vi "Vending Machine.vi"() -> ()   [LabVIEW 2016]
panel:
  in  "반환":bool
  out "거스름돈":string
  out "백원 갯수":string
  out "오백원 갯수":string
  in  "500원권":bool
  out "파워":dbl(slide)
  out "비타민":dbl(slide)
  out "파워에이드 재고":string
  out "비타민 워터 재고":string
  out "사이다 재고":string
  out "콜라 재고":string
  out "Display \nMoney":dbl
  out "사이다 뽑음":dbl(slide)
  in  "100원권":bool
  in  "1000원권":bool
  in  "5000원권":bool
  in  "10000원권":bool
  in  "카드":bool
  in  "2000 원":bool
  in  "1500 원":bool
  in  "1000 원":bool
  in  "700 원":bool
  in  "자판기 멈춤":bool
  out "콜라뽑음":dbl(slide)
  # "27기 인턴 \n 하 유 진"
  # "원"
  # "거스름 동전 재고"
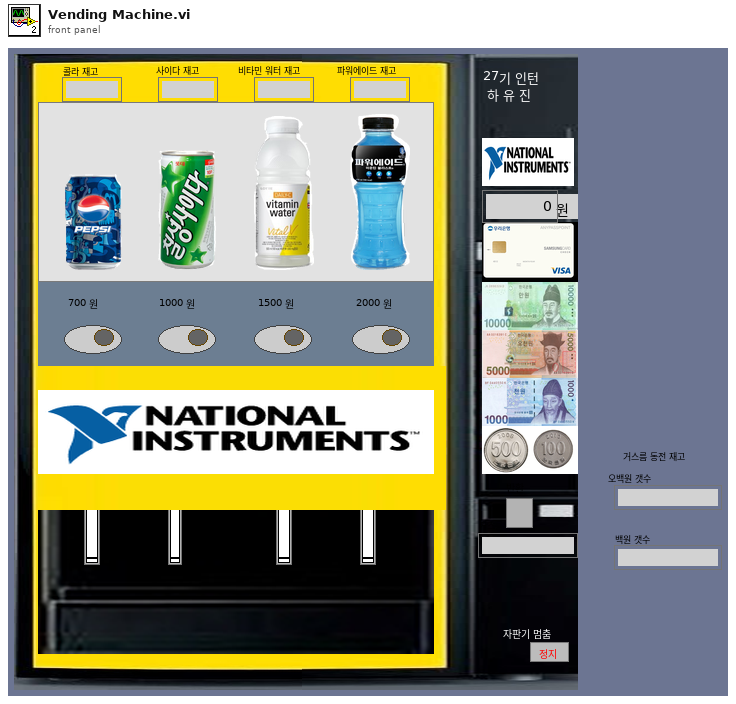
[diagram p1: front panel]
types:
  T1 = cluster{"재고1":i32, "재고2":i32, "재고3":i32, "재고4":i32}
  T2 = cluster{"700원":bool, " 1000원":bool, "1500원":bool, "2000원":bool}
  T3 = cluster{"10000":bool, " 5000":bool, "1000":bool, "100":bool, "500":bool, "카드":bool}
  T4 = typedef "컨트롤 3.ctl" = enum32{"대기", "돈 투입", "돈 반환", "음료 재고", "음료 주문", "카드"}
  T5 = enum16{"대기", "돈 투입", "돈 반환", "음료 재고", "음료 주문", "카드"}
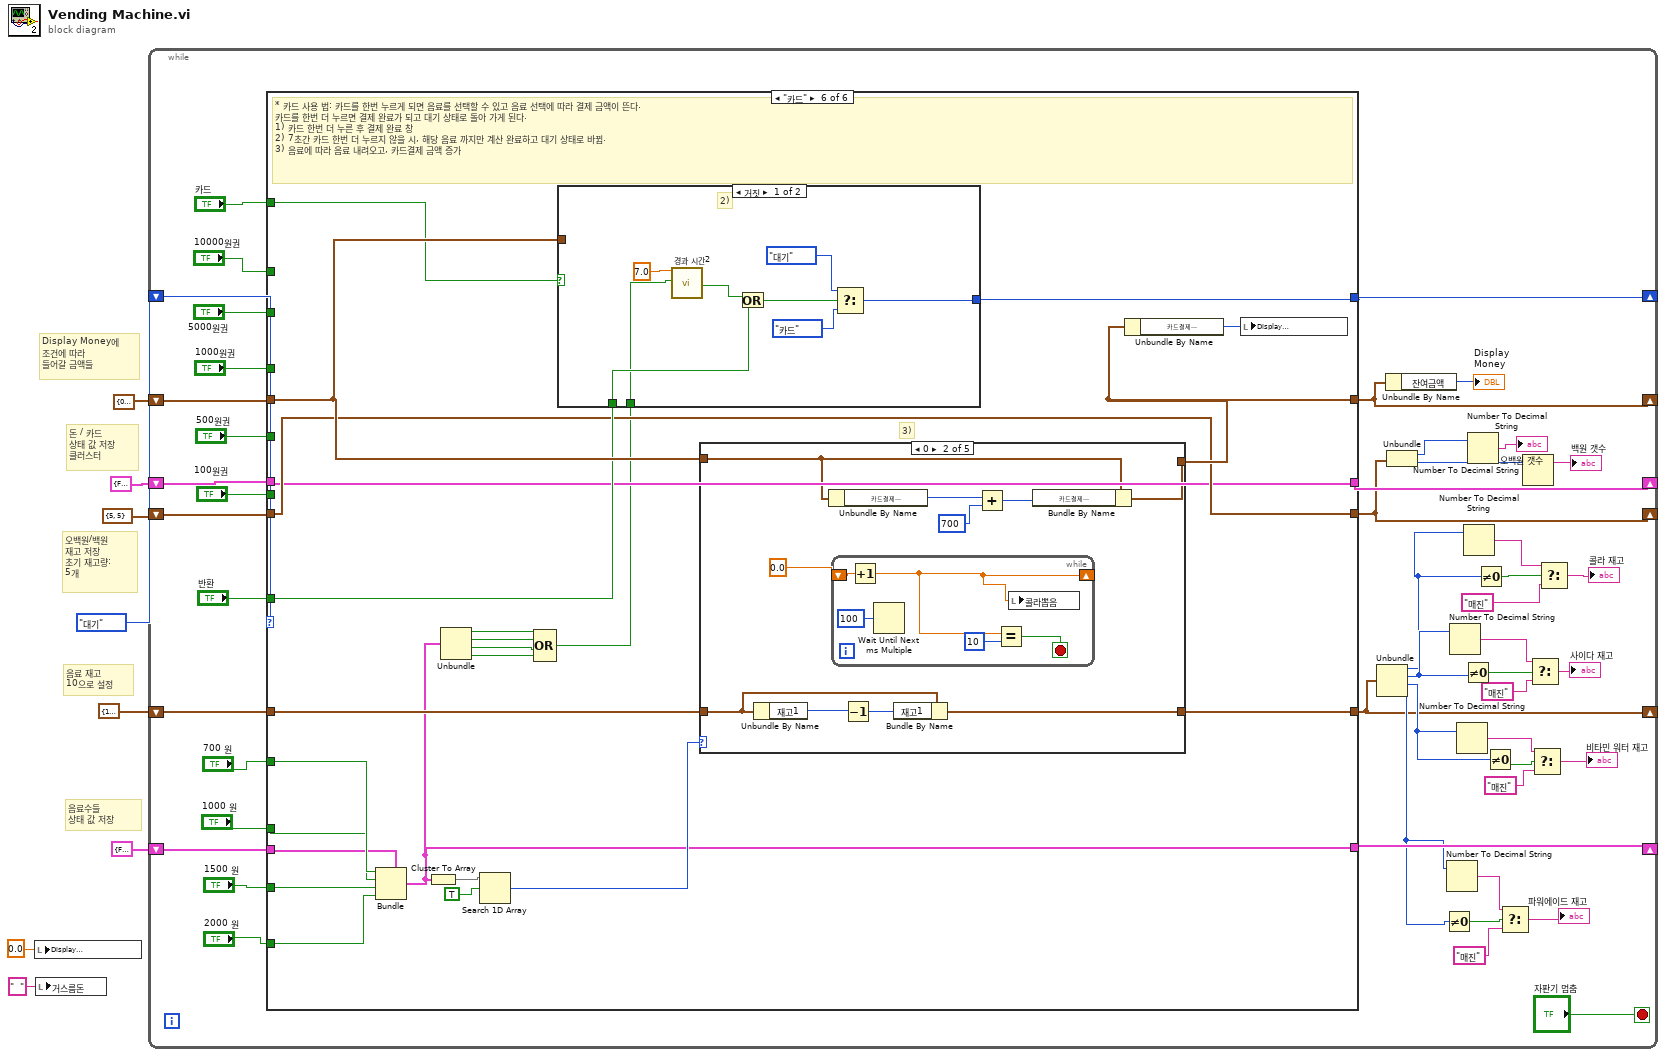
[diagram p0: block diagram]
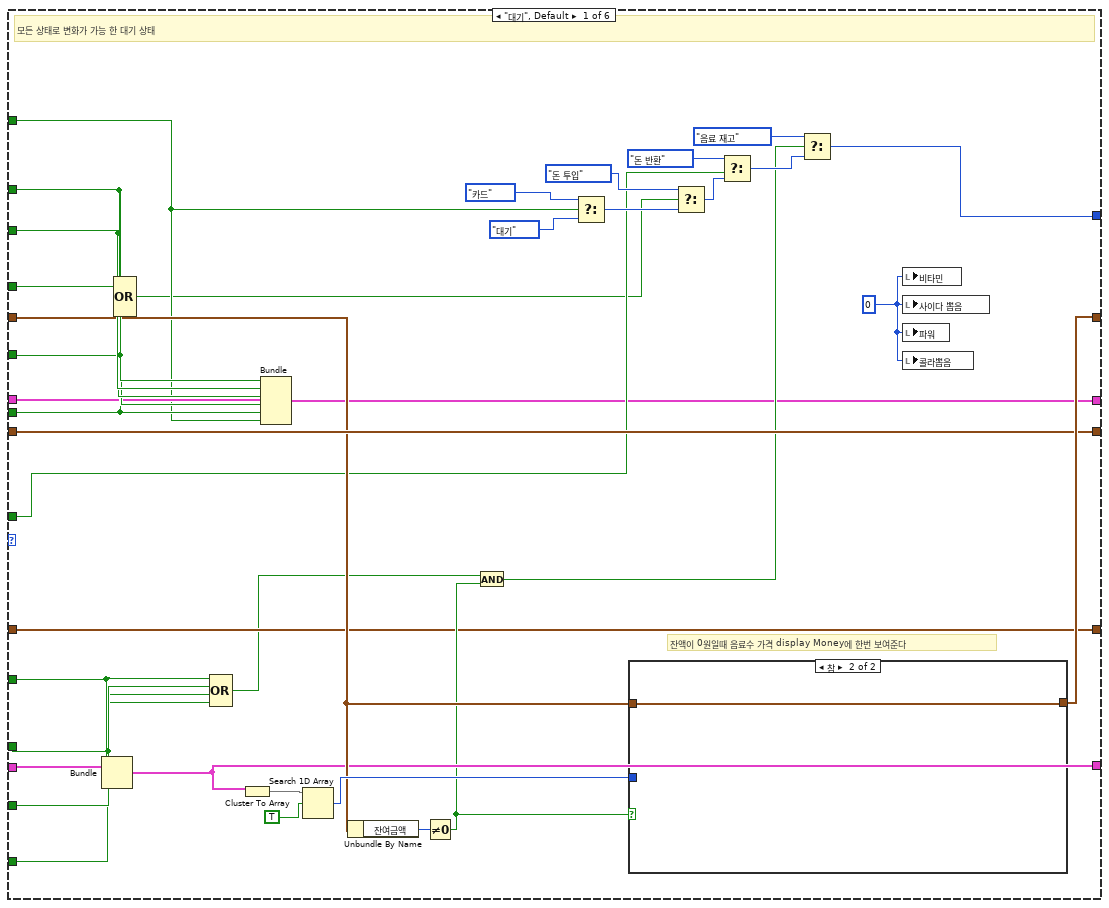
[diagram p2: hidden frame]
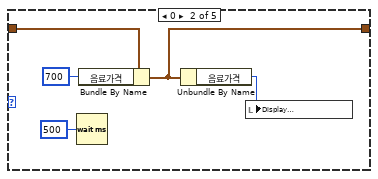
[diagram p4: hidden frame]
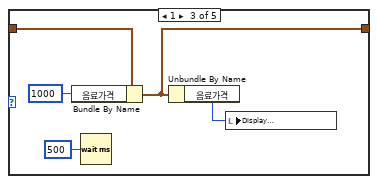
[diagram p5: hidden frame]
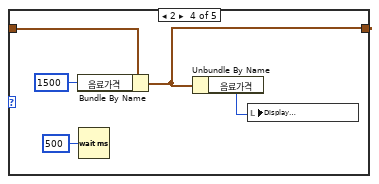
[diagram p6: hidden frame]
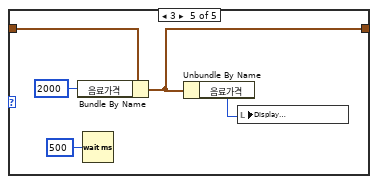
[diagram p7: hidden frame]
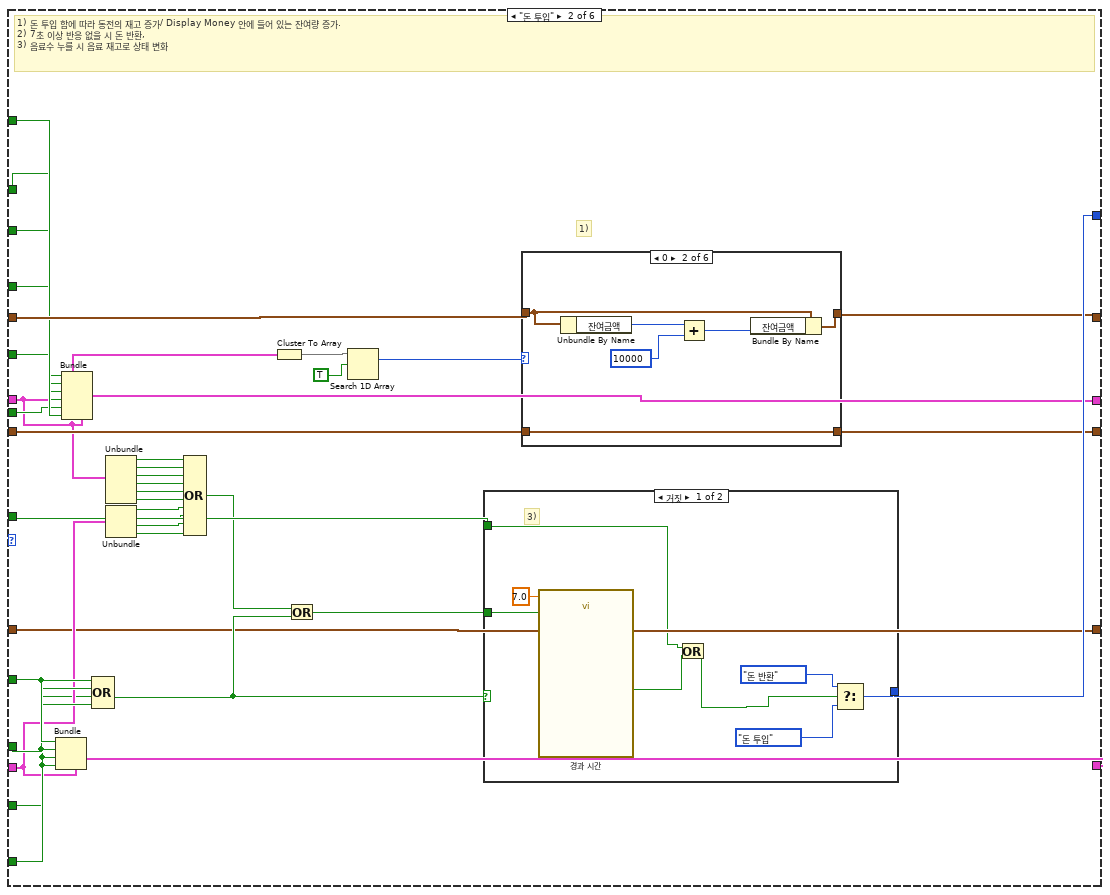
[diagram p8: hidden frame]
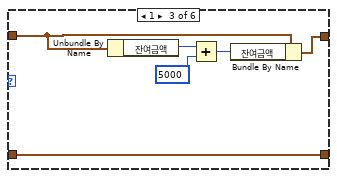
[diagram p10: hidden frame]
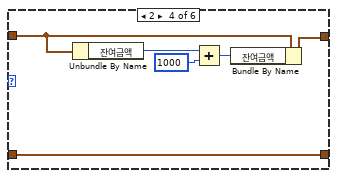
[diagram p11: hidden frame]
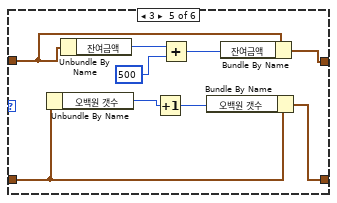
[diagram p12: hidden frame]
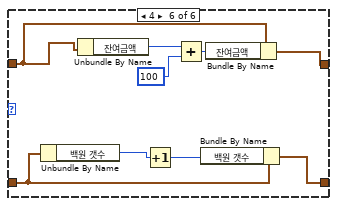
[diagram p13: hidden frame]
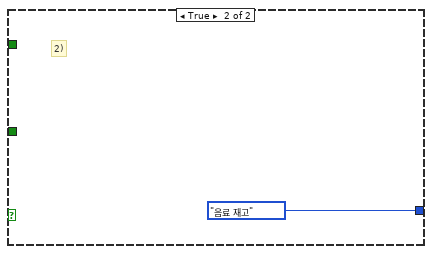
[diagram p14: hidden frame]
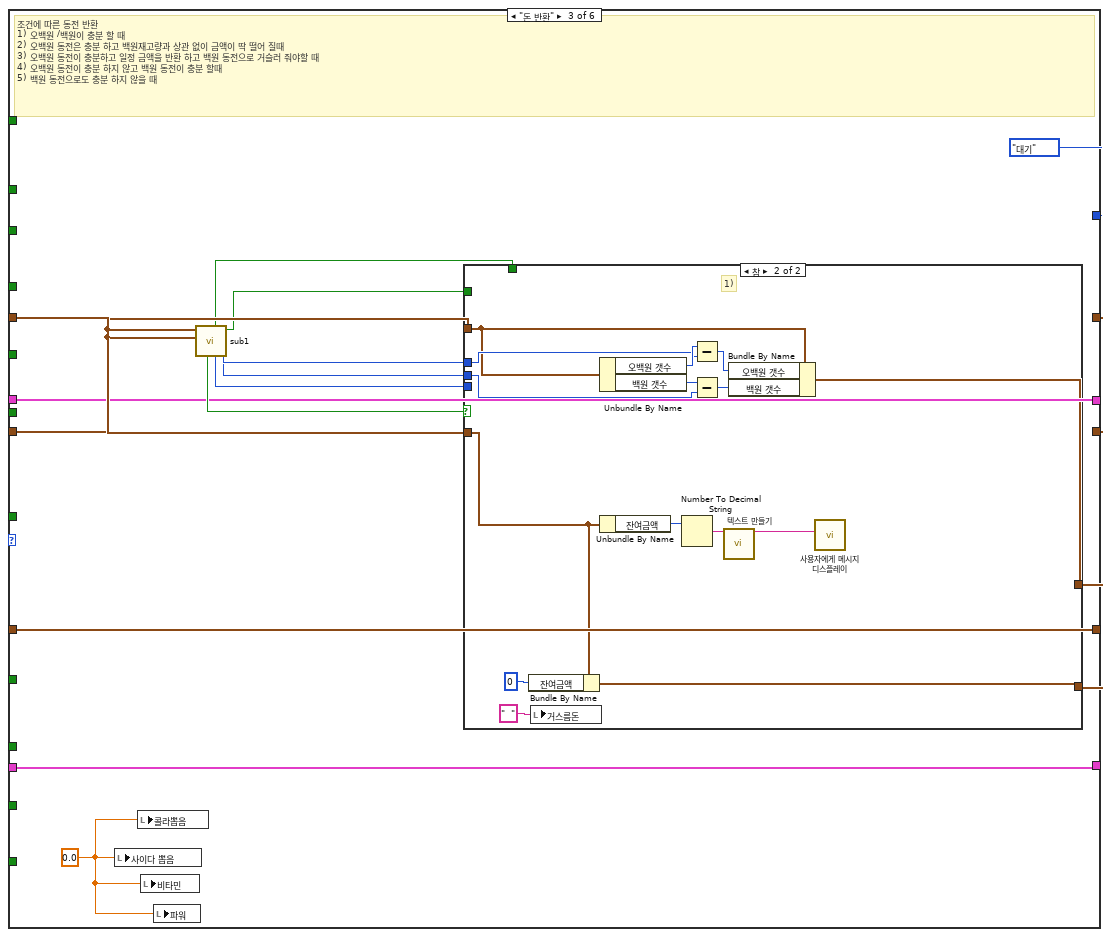
[diagram p15: hidden frame]
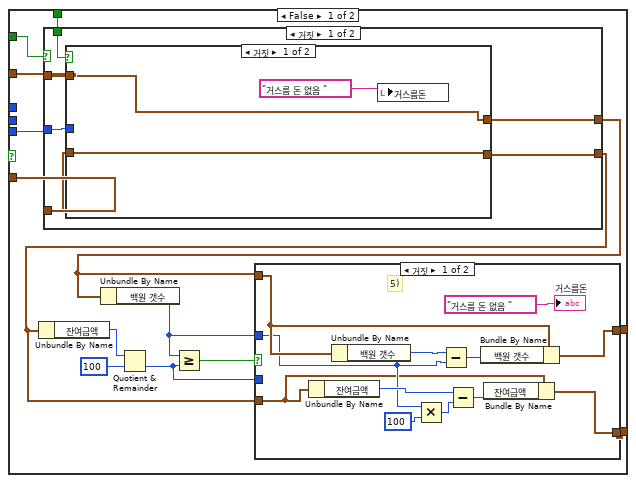
[diagram p16: hidden frame]
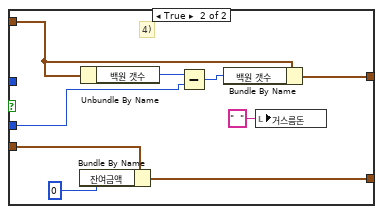
[diagram p17: hidden frame]
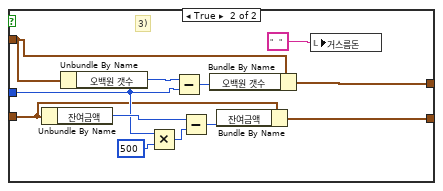
[diagram p18: hidden frame]
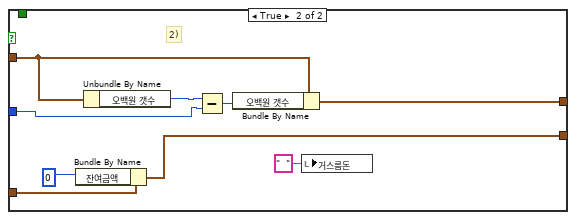
[diagram p19: hidden frame]
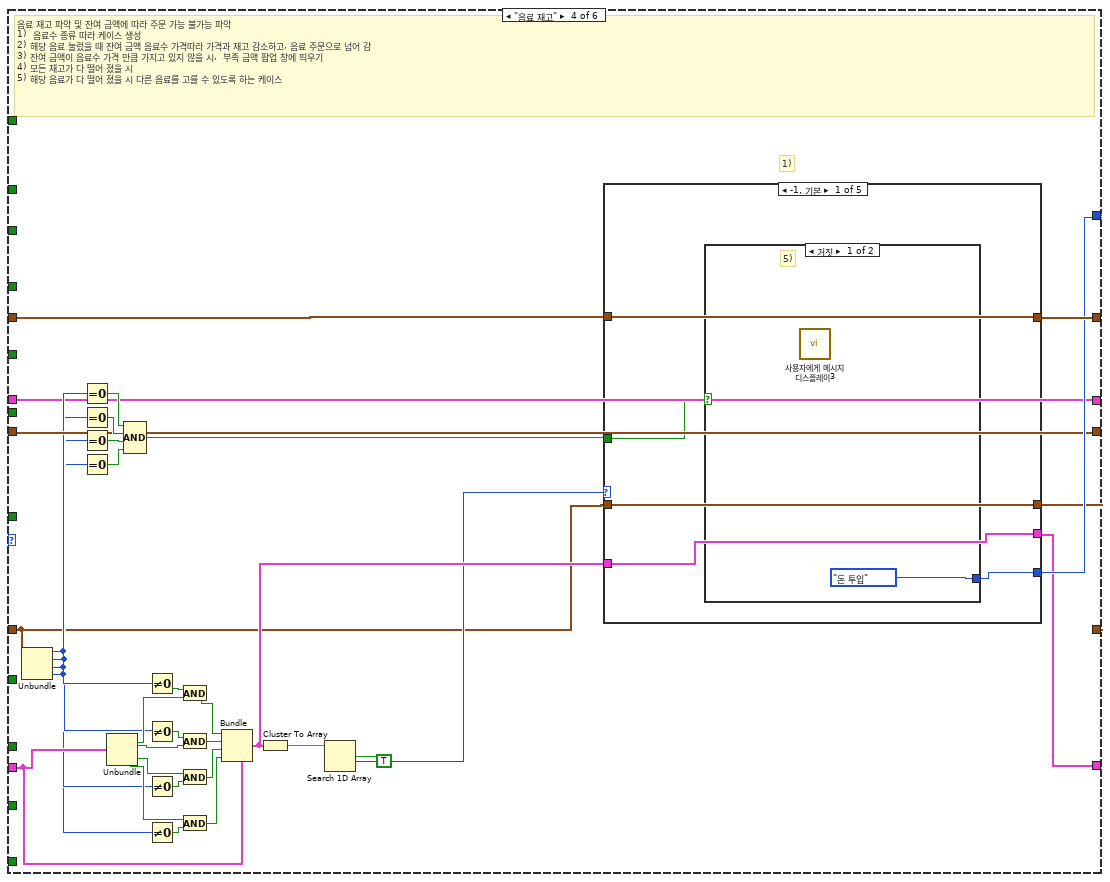
[diagram p20: hidden frame]
diagram:
  # "음료 재고 \n10으로 설정"
  # "음료수들  \n상태 값 저장"
  # "오백원/백원\n재고 저장\n초기 재고량: \n5개"
  # "돈 / 카드 \n상태 값 저장\n클러스터"
  # "Display Money에 \n조건에 따라\n들어갈 금액들"
  n1 = local write "Display \nMoney"(0.0 ("Display \nMoney")) -> ()
  n2 = local write "거스름돈"("  " ("거스름돈")) -> ()
  n3 = while {
    shift-right: [w50] -> _
    shift-left: 컨트롤_3."대기" -> [w39]
    shift-right: [w42] -> _
    shift-left: cluster{"잔여금액":i32, "카드결제\n금액":i32, "음료가격":i32} {"잔여금액"=0, "카드결제\n금액"=0, "음료가격"=0} -> [w45]
    shift-right: [w44] -> _
    shift-left: T3 {"10000"=FALSE, " 5000"=FALSE, "1000"=FALSE, "100"=FALSE, "500"=FALSE, "카드"=FALSE} -> [w38]
    shift-right: [w40] -> _
    shift-left: T2 {"700원"=FALSE, " 1000원"=FALSE, "1500원"=FALSE, "2000원"=FALSE} -> [w43]
    shift-right: [w10] -> _
    shift-left: cluster{"오백원 갯수":i32, " 백원 갯수":i32} {"오백원 갯수"=5, " 백원 갯수"=5} -> [w24]
    shift-right: [w13] -> _
    shift-left: T1 {"재고1"=10, "재고2"=10, "재고3"=10, "재고4"=10} -> [w19]
    stop <- "자판기 멈춤" stop-if-true
    n4 = case shown="\"카드\"" w39 {
      tunnel: "카드" -> [w72 w146 _ _ _ w519]
      tunnel: "10000원권" -> [w94 w142 _ _ _ _]
      tunnel: "5000원권" -> [w93 w141 _ _ _ _]
      tunnel: "1000원권" -> [w92 w140 _ _ _ _]
      tunnel: "500원권" -> [w91 w139 _ _ _ _]
      tunnel: "100원권" -> [w90 w138 _ _ _ _]
      tunnel: [w65 w156 T5."대기" w314 w468 w525] -> w50
      tunnel: "700 원" -> [w80 w155 _ _ _ w534]
      tunnel: "1000 원" -> [w79 w154 _ _ _ w533]
      tunnel: "1500 원" -> [w78 w120 _ _ _ w532]
      tunnel: "2000 원" -> [w77 w153 _ _ _ w531]
      tunnel: w45 -> [w81 w148 w217 w315 w480 w527]
      tunnel: [w85 w147 w206 w317 w480 w524] -> w42
      tunnel: w38 -> [w84 w135 w204 w300 w483 w518]
      tunnel: [w61 w121 w204 w300 w483 w518] -> w44
      tunnel: w43 -> [w86 w128 w205 w324 w482 w517]
      tunnel: [w76 w152 w205 w299 w482 w516] -> w40
      tunnel: "반환" -> [w63 w145 _ _ w474 w526]
      tunnel: w24 -> [w82 w144 w215 w307 w481 w522]
      tunnel: [w82 w143 w216 w307 w481 w522] -> w10
      tunnel: w19 -> [w59 w122 w207 w302 w478 w521]
      tunnel: [w59 w122 w207 w301 w478 w520] -> w13
      frame "대기", Default {
        w83 = 0
        # "잔액이 0원일때 음료수 가격 display Money에 한번 보여준다"
        # "모든 상태로 변화가 가능 한 대기 상태"
        n5 = Bundle(cluster=w86, "700원"=w80, "1000원"=w79, "1500원"=w78, "2000원"=w77) -> (w76:T2)
        n6 = Compound Arithmetic op=OR ("복합 연산")(w94, w93, w92, w91, w90) -> (w62:bool)
        n7 = Compound Arithmetic op=OR ("복합 연산")(w80, w79, w78, w77) -> (w58:bool)
        n8 = Cluster To Array(cluster=w76) -> (array=w89:bool[])
        n9 = Bundle(cluster=w84, "10000"=w94, "5000"=w93, "1000"=w92, "100"=w91, "500"=w90, "카드"=w72) -> (w61:T3)
        n10 = Search 1D Array(1D array=w89, element=TRUE ("원소")) -> (index of element=w88:i32)  [unwired: 1 in]
        n11 = Unbundle By Name(w81) -> ("잔여금액"=w60:i32)
        n12 = Not Equal To 0?(x=w60) -> (x != 0?=w75:bool)
        n13 = And(x=w58, y=w75) -> (x .and. y?=w67:bool)
        n14 = Select(t=T5."카드", s=w72, f=T5."대기") -> (s? t:f=w71:T5)
        n15 = case shown="참" w75 {
          tunnel: w88 -> [w97 _]
          tunnel: [w96 w119] -> w85
          tunnel: w81 -> [w95 w119]
          frame False {
            n16 = case shown="-1, 기본" w97 {
              tunnel: w95 -> [w98 w103 w107 w112 w117]
              tunnel: [w98 w101 w105 w110 w115] -> w96
              frame -1, Default {
              }
              frame 0 {
                n17 = Wait (ms)(milliseconds to wait=u32 500 ("대기 시간 (ms)")) -> ()  [unwired: 1 out]
                n18 = Bundle By Name(cluster=w103, "음료가격"=700 ("잔여금액")) -> (w101:cluster{"잔여금액":i32, "카드결제\n금액":i32, "음료가격":i32})
                n19 = Unbundle By Name(w101) -> ("음료가격"=w100:i32)
                n20 = local write "Display \nMoney"(w100) -> ()
              }
              frame 1 {
                n21 = Bundle By Name(cluster=w107, "음료가격"=1000 ("잔여금액")) -> (w105:cluster{"잔여금액":i32, "카드결제\n금액":i32, "음료가격":i32})
                n22 = Wait (ms)(milliseconds to wait=u32 500 ("대기 시간 (ms)")) -> ()  [unwired: 1 out]
                n23 = Unbundle By Name(w105) -> ("음료가격"=w106:i32)
                n24 = local write "Display \nMoney"(w106) -> ()
              }
              frame 2 {
                n25 = Bundle By Name(cluster=w112, "음료가격"=1500 ("잔여금액")) -> (w110:cluster{"잔여금액":i32, "카드결제\n금액":i32, "음료가격":i32})
                n26 = Wait (ms)(milliseconds to wait=u32 500 ("대기 시간 (ms)")) -> ()  [unwired: 1 out]
                n27 = Unbundle By Name(w110) -> ("음료가격"=w111:i32)
                n28 = local write "Display \nMoney"(w111) -> ()
              }
              frame 3 {
                n29 = Bundle By Name(cluster=w117, "음료가격"=2000 ("잔여금액")) -> (w115:cluster{"잔여금액":i32, "카드결제\n금액":i32, "음료가격":i32})
                n30 = Wait (ms)(milliseconds to wait=u32 500 ("대기 시간 (ms)")) -> ()  [unwired: 1 out]
                n31 = Unbundle By Name(w115) -> ("음료가격"=w116:i32)
                n32 = local write "Display \nMoney"(w116) -> ()
              }
            }
          }
          frame True {
          }
        }
        n33 = Select(t=T5."돈 투입", s=w62, f=w71) -> (s? t:f=w69:T5)
        n34 = Select(t=T5."돈 반환", s=w63, f=w69) -> (s? t:f=w68:T5)
        n35 = Select(t=T5."음료 재고", s=w67, f=w68) -> (s? t:f=w65:T5)
        n36 = local write "비타민"(w83) -> ()
        n37 = local write "사이다 뽑음"(w83) -> ()
        n38 = local write "파워"(w83) -> ()
        n39 = local write "콜라뽑음"(w83) -> ()
      }
      frame "돈 투입" {
        # "1)"
        # "1) 돈 투입 함에 따라 동전의 재고 증가/ Display Money 안에 들어 있는 잔여량 증가.\n2) 7초 이상 반응 없을 시 돈 반환, \n3) 음료수 누를 시 음료 재고로 상태 변화"
        n40 = Bundle(cluster=w128, "700원"=w155, "1000원"=w154, "1500원"=w120, "2000원"=w153) -> (w152:T2)
        n41 = Bundle(cluster=w135, "10000"=w142, "5000"=w141, "1000"=w140, "100"=w139, "500"=w138, "카드"=w146) -> (w121:T3)
        n42 = Compound Arithmetic op=OR ("복합 연산")(w155, w154, w120, w153) -> (w123:bool)
        n43 = Unbundle(w135) -> ("10000"=w134:bool, "5000"=w133:bool, "1000"=w132:bool, "100"=w131:bool, "500"=w130:bool, "카드"=w129:bool)
        n44 = Unbundle(w128) -> ("700원"=w127:bool, "1000원"=w126:bool, "1500원"=w125:bool, "2000원"=w124:bool)
        n45 = Compound Arithmetic op=OR ("복합 연산")(w134, w133, w132, w131, w130, w129, w127, w126, w125, w124) -> (w137:bool)
        n46 = Cluster To Array(cluster=w135) -> (array=w151:bool[])
        n47 = Or(x=w137, y=w123) -> (x .or. y?=w136:bool)
        n48 = Search 1D Array(1D array=w151, element=TRUE ("원소")) -> (index of element=w149:i32)  [unwired: 1 in]
        n49 = case shown="거짓" w123 {
          tunnel: [w201 T5."음료 재고"] -> w156
          tunnel: w145 -> [w199 _]
          tunnel: w136 -> [w195 _]
          frame False {
            # "3)"
            n50 = call "경과 시간"("Time Target (s)"=7.0, "Reset"=w195) -> ("Time has Elapsed"=w196:bool)  [unwired: 10 in, 7 out]
            n51 = Or(x=w199, y=w196) -> (x .or. y?=w198:bool)
            n52 = Select(t=T5."돈 반환", s=w198, f=T5."돈 투입") -> (s? t:f=w201:T5)
          }
          frame True {
            # "2)"
          }
        }
        n53 = case shown="0" w149 {
          tunnel: w148 -> [w158 w161 w167 w173 w182 w191]
          tunnel: [w158 w160 w166 w172 w181 w190] -> w147
          tunnel: w144 -> [w157 w159 w165 w171 w179 w187]
          tunnel: [w157 w159 w165 w171 w178 w186] -> w143
          frame -1, Default {
          }
          frame 0 {
            n54 = Unbundle By Name(w161) -> ("잔여금액"=w162:i32)
            n55 = Add(x=w162, y=10000) -> (x+y=w164:i32)
            n56 = Bundle By Name(cluster=w161, "잔여금액"=w164) -> (w160:cluster{"잔여금액":i32, "카드결제\n금액":i32, "음료가격":i32})
          }
          frame 1 {
            n57 = Unbundle By Name(w167) -> ("잔여금액"=w168:i32)
            n58 = Add(x=w168, y=5000) -> (x+y=w169:i32)
            n59 = Bundle By Name(cluster=w167, "잔여금액"=w169) -> (w166:cluster{"잔여금액":i32, "카드결제\n금액":i32, "음료가격":i32})
          }
          frame 2 {
            n60 = Unbundle By Name(w173) -> ("잔여금액"=w174:i32)
            n61 = Add(x=w174, y=1000) -> (x+y=w176:i32)
            n62 = Bundle By Name(cluster=w173, "잔여금액"=w176) -> (w172:cluster{"잔여금액":i32, "카드결제\n금액":i32, "음료가격":i32})
          }
          frame 3 {
            n63 = Unbundle By Name(w179) -> ("오백원 갯수"=w177:i32)
            n64 = Unbundle By Name(w182) -> ("잔여금액"=w184:i32)
            n65 = Increment(x=w177) -> (x+1=w180:i32)
            n66 = Add(x=w184, y=500) -> (x+y=w185:i32)
            n67 = Bundle By Name(cluster=w179, "오백원 갯수"=w180) -> (w178:cluster{"오백원 갯수":i32, " 백원 갯수":i32})
            n68 = Bundle By Name(cluster=w182, "잔여금액"=w185) -> (w181:cluster{"잔여금액":i32, "카드결제\n금액":i32, "음료가격":i32})
          }
          frame 4 {
            n69 = Unbundle By Name(w187) -> ("백원 갯수"=w188:i32)
            n70 = Unbundle By Name(w191) -> ("잔여금액"=w192:i32)
            n71 = Increment(x=w188) -> (x+1=w189:i32)
            n72 = Add(x=w192, y=100) -> (x+y=w194:i32)
            n73 = Bundle By Name(cluster=w187, "백원 갯수"=w189) -> (w186:cluster{"오백원 갯수":i32, " 백원 갯수":i32})
            n74 = Bundle By Name(cluster=w191, "잔여금액"=w194) -> (w190:cluster{"잔여금액":i32, "카드결제\n금액":i32, "음료가격":i32})
          }
        }
      }
      frame "돈 반환" {
        w208 = 0.0 ("사이다 뽑힘")
        # "조건에 따른 동전 반환 \n1) 오백원 /백원이 충분 할 때\n2) 오백원 동전은 충분 하고 백원재고량과 상관 없이 금액이 딱 떨어 질때\n3) 오백원 동전이 충분하고 일정 금액을 반환 하고 백원 동전으로 거슬러 줘야할 때 \n4) 오백원 동전이 충분 하지 않고 백원 동전이 충분 할때\n5) 백원 동전으로도 충분 하지 않을 때"
        n75 = local write "사이다 뽑음"(w208) -> ()
        n76 = local write "콜라뽑음"(w208) -> ()
        n77 = local write "비타민"(w208) -> ()
        n78 = local write "파워"(w208) -> ()
        n79 = call "sub1.vi"("클러스터"=w215, "클러스터 2"=w217) -> ("숫자형"=w212:i32, "숫자형 2"=w213:i32, "불리언 2"=w210:bool, "오백원 갯수"=w211:i32, "불리언"=w209:bool, "불리언 3"=w214:bool)  [unwired: 4 in]
        n80 = case shown="참" w214 {
          tunnel: w215 -> [w231 w296]
          tunnel: w213 -> [_ w297]
          tunnel: w212 -> [_ w293]
          tunnel: w210 -> [w232 _]
          tunnel: w217 -> [w230 w287]
          tunnel: w211 -> [w229 _]
          tunnel: [w223 w286] -> w206
          tunnel: [w222 w285] -> w216
          tunnel: w209 -> [w219 _]
          frame False {
            n81 = case shown="거짓" w232 {
              tunnel: w231 -> [w259 w279]
              tunnel: [w258 w282] -> w225
              tunnel: w229 -> [w257 w281]
              tunnel: w230 -> [w256 w277]
              tunnel: [w255 w276] -> w224
              tunnel: w219 -> [w254 _]
              frame False {
                n82 = case shown="거짓" w254 {
                  tunnel: w259 -> [w261 w272]
                  tunnel: [w261 w271] -> w258
                  tunnel: w257 -> [_ w269]
                  tunnel: w256 -> [w260 w267]
                  tunnel: [w260 w265] -> w255
                  frame False {
                    n83 = local write "거스름돈"("거스름 돈 없음 " ("거스름돈")) -> ()
                  }
                  frame True {
                    # "3)"
                    n84 = Unbundle By Name(w267) -> ("잔여금액"=w270:i32)
                    n85 = Unbundle By Name(w272) -> ("오백원 갯수"=w273:i32)
                    n86 = Multiply(x=w269, y=500) -> (x*y=w264:i32)
                    n87 = Subtract(x=w273, y=w269) -> (x-y=w274:i32)
                    n88 = Subtract(x=w270, y=w264) -> (x-y=w266:i32)
                    n89 = Bundle By Name(cluster=w272, "오백원 갯수"=w274) -> (w271:cluster{"오백원 갯수":i32, " 백원 갯수":i32})
                    n90 = Bundle By Name(cluster=w267, "잔여금액"=w266) -> (w265:cluster{"잔여금액":i32, "카드결제\n금액":i32, "음료가격":i32})
                    n91 = local write "거스름돈"("   " ("거스름돈")) -> ()
                  }
                }
              }
              frame True {
                # "2)"
                n92 = Bundle By Name(cluster=w277, "잔여금액"=0) -> (w276:cluster{"잔여금액":i32, "카드결제\n금액":i32, "음료가격":i32})
                n93 = Unbundle By Name(w279) -> ("오백원 갯수"=w280:i32)
                n94 = Subtract(x=w280, y=w281) -> (x-y=w283:i32)
                n95 = Bundle By Name(cluster=w279, "오백원 갯수"=w283) -> (w282:cluster{"오백원 갯수":i32, " 백원 갯수":i32})
                n96 = local write "거스름돈"("  " ("거스름돈")) -> ()
              }
            }
            n97 = Unbundle By Name(w224) -> ("잔여금액"=w227:i32)
            n98 = Unbundle By Name(w225) -> ("백원 갯수"=w221:i32)
            n99 = Quotient & Remainder(x=w227, y=100) -> (floor(x/y)=w220:i32)  [unwired: 1 out]
            n100 = Greater Or Equal?(x=w221, y=w220) -> (x >= y?=w228:bool)
            n101 = case shown="거짓" w228 {
              tunnel: w225 -> [w237 w250]
              tunnel: w224 -> [w235 w249]
              tunnel: w220 -> [_ w248]
              tunnel: [w234 w247] -> w223
              tunnel: [w233 w246] -> w222
              tunnel: w221 -> [w236 _]
              frame False {
                # "5)"
                n102 = Unbundle By Name(w235) -> ("잔여금액"=w241:i32)
                n103 = Unbundle By Name(w237) -> ("백원 갯수"=w242:i32)
                n104 = Multiply(x=w236, y=100) -> (x*y=w238:i32)
                n105 = Subtract(x=w242, y=w236) -> (x-y=w243:i32)
                n106 = Subtract(x=w241, y=w238) -> (x-y=w239:i32)
                n107 = Bundle By Name(cluster=w237, "백원 갯수"=w243) -> (w233:cluster{"오백원 갯수":i32, " 백원 갯수":i32})
                n108 = Bundle By Name(cluster=w235, "잔여금액"=w239) -> (w234:cluster{"잔여금액":i32, "카드결제\n금액":i32, "음료가격":i32})
                "거스름돈" <- "거스름 돈 없음 " ("거스름돈")
              }
              frame True {
                # "4)"
                n109 = Bundle By Name(cluster=w249, "잔여금액"=0) -> (w247:cluster{"잔여금액":i32, "카드결제\n금액":i32, "음료가격":i32})
                n110 = Unbundle By Name(w250) -> ("백원 갯수"=w253:i32)
                n111 = Subtract(x=w253, y=w248) -> (x-y=w252:i32)
                n112 = Bundle By Name(cluster=w250, "백원 갯수"=w252) -> (w246:cluster{"오백원 갯수":i32, " 백원 갯수":i32})
                n113 = local write "거스름돈"("  " ("거스름돈")) -> ()
              }
            }
          }
          frame True {
            # "1)"
            n114 = Bundle By Name(cluster=w287, "잔여금액"=0) -> (w286:cluster{"잔여금액":i32, "카드결제\n금액":i32, "음료가격":i32})
            n115 = local write "거스름돈"("  " ("거스름돈")) -> ()
            n116 = Unbundle By Name(w296) -> ("오백원 갯수"=w298:i32, "백원 갯수"=w294:i32)
            n117 = Unbundle By Name(w287) -> ("잔여금액"=w289:i32)
            n118 = Number To Decimal String(number=w289) -> (decimal integer string=w291:string)  [unwired: 1 in]
            n119 = Subtract(x=w298, y=w297) -> (x-y=w295:i32)
            n120 = Subtract(x=w294, y=w293) -> (x-y=w292:i32)
            n121 = call "텍스트 만들기"("Beginning Text"=w291) -> ("Result"=w290:string)  [unwired: 13 in, 1 out]
            n122 = Bundle By Name(cluster=w296, "오백원 갯수"=w295, "백원 갯수"=w292) -> (w285:cluster{"오백원 갯수":i32, " 백원 갯수":i32})
            n123 = call "사용자에게 메시지 디스플레이"("Message"=w290) -> ()  [unwired: 9 in, 2 out]
          }
        }
      }
      frame "음료 재고" {
        # "1)"
        # "음료 재고 파악 및 잔여 금액에 따라 주문 가능 불가능 파악\n1)  음료수 종류 따라 케이스 생성\n2) 해당 음료 눌렀을 때 잔여 금액 음료수 가격따라 가격과 재고 감소하고, 음료 주문으로 넘어 감\n3) 잔여 금액이 음료수 가격 만큼 가지고 있지 않을 시,  부족 금액 팝업 창에 띄우기 \n4) 모든 재고가 다 떨어 졌을 시 \n5) 해당 음료가 다 떨어 졌을 시 다른 음료를 고를 수 있도록 하는 케이스"
        n124 = Unbundle(w302) -> ("재고1"=w306:i32, "재고2"=w305:i32, "재고3"=w304:i32, "재고4"=w303:i32)
        n125 = Equal To 0?(x=w306) -> (x = 0?=w312:bool)
        n126 = Equal To 0?(x=w305) -> (x = 0?=w311:bool)
        n127 = Equal To 0?(x=w304) -> (x = 0?=w310:bool)
        n128 = Equal To 0?(x=w303) -> (x = 0?=w309:bool)
        n129 = Unbundle(w324) -> ("700원"=w332:bool, "1000원"=w331:bool, "1500원"=w330:bool, "2000원"=w329:bool)
        n130 = Compound Arithmetic op=AND ("복합 연산")(w312, w311, w310, w309) -> (w308:bool)
        n131 = Not Equal To 0?(x=w306) -> (x != 0?=w328:bool)
        n132 = Not Equal To 0?(x=w305) -> (x != 0?=w325:bool)
        n133 = Not Equal To 0?(x=w304) -> (x != 0?=w326:bool)
        n134 = Not Equal To 0?(x=w303) -> (x != 0?=w327:bool)
        n135 = And(x=w328, y=w332) -> (x .and. y?=w323:bool)
        n136 = And(x=w325, y=w331) -> (x .and. y?=w322:bool)
        n137 = And(x=w330, y=w326) -> (x .and. y?=w321:bool)
        n138 = And(x=w329, y=w327) -> (x .and. y?=w320:bool)
        n139 = Bundle(cluster=w324, "700원"=w323, "1000원"=w322, "1500원"=w321, "2000원"=w320) -> (w316:T2)
        n140 = Cluster To Array(cluster=w316) -> (array=w319:bool[])
        n141 = Search 1D Array(1D array=w319, element=TRUE ("원소")) -> (index of element=w313:i32)  [unwired: 1 in]
        n142 = case shown="-1, 기본" w313 {
          tunnel: w315 -> [w335 w345 w376 w407 w439]
          tunnel: [w335 w349 w381 w406 w445] -> w317
          tunnel: w316 -> [w336 w348 w379 w412 w443]
          tunnel: [w336 w347 w378 w411 w442] -> w299
          tunnel: [w337 w346 w380 w413 w444] -> w314
          tunnel: w308 -> [w334 _ _ _ _]
          tunnel: w302 -> [w333 w341 w373 w405 w437]
          tunnel: [w333 w340 w372 w404 w436] -> w301
          frame -1, Default {
            n143 = case shown="거짓" w334 {
              tunnel: [T5."돈 투입" T5."돈 반환"] -> w337
              frame False {
                # "5)"
                n144 = call "사용자에게 메시지 디스플레이3"() -> ()  [unwired: 10 in, 2 out]
              }
              frame True {
                # "4)"
                n145 = call "사용자에게 메시지 디스플레이2"() -> ()  [unwired: 10 in, 2 out]
              }
            }
          }
          frame 0 {
            n146 = Unbundle By Name(w345) -> ("잔여금액"=w344:i32)
            n147 = Greater Or Equal?(x=w344, y=700) -> (x >= y?=w342:bool)
            n148 = case shown="거짓" w342 {
              tunnel: w345 -> [w356 w368]
              tunnel: [w356 w367] -> w349
              tunnel: w348 -> [w357 w366]
              tunnel: [w357 w364] -> w347
              tunnel: [T5."대기" T5."음료 주문"] -> w346
              tunnel: w341 -> [w350 w359]
              tunnel: [w350 w360] -> w340
              frame False {
                # "3)"
                n149 = Unbundle By Name(w356) -> ("잔여금액"=w355:i32)
                n150 = Subtract(x=700, y=w355) -> (x-y=w353:i32)
                n151 = Number To Decimal String(number=w353) -> (decimal integer string=w352:string)  [unwired: 1 in]
                n152 = call "텍스트 만들기3"("Beginning Text"=w352) -> ("Result"=w351:string)  [unwired: 13 in, 1 out]
                n153 = call "사용자에게 메시지 디스플레이4"("Message"=w351) -> ()  [unwired: 9 in, 2 out]
              }
              frame True {
                # "2)"
                n154 = Unbundle By Name(w368) -> ("잔여금액"=w369:i32)
                n155 = Unbundle By Name(w359) -> ("재고1"=w362:i32)
                n156 = Bundle By Name(cluster=w366, "700원"=TRUE) -> (w364:T2)
                n157 = Decrement(x=w362) -> (x-1=w361:i32)
                n158 = Subtract(x=w369, y=700) -> (x-y=w371:i32)
                n159 = Bundle By Name(cluster=w368, "잔여금액"=w371) -> (w367:cluster{"잔여금액":i32, "카드결제\n금액":i32, "음료가격":i32})
                n160 = Bundle By Name(cluster=w359, "재고1"=w361) -> (w360:T1)
              }
            }
          }
          frame 1 {
            n161 = Unbundle By Name(w376) -> ("잔여금액"=w375:i32)
            n162 = Greater Or Equal?(x=w375, y=1000) -> (x >= y?=w374:bool)
            n163 = case shown="거짓" w374 {
              tunnel: w376 -> [w385 w400]
              tunnel: [w385 w399] -> w381
              tunnel: [T5."대기" T5."음료 주문"] -> w380
              tunnel: w379 -> [w389 w397]
              tunnel: [w389 w395] -> w378
              tunnel: w373 -> [w382 w392]
              tunnel: [w382 w391] -> w372
              frame False {
                n164 = Unbundle By Name(w385) -> ("잔여금액"=w388:i32)
                n165 = Subtract(x=1000, y=w388) -> (x-y=w386:i32)
                n166 = Number To Decimal String(number=w386) -> (decimal integer string=w383:string)  [unwired: 1 in]
                n167 = call "텍스트 만들기4"("Beginning Text"=w383) -> ("Result"=w384:string)  [unwired: 13 in, 1 out]
                n168 = call "사용자에게 메시지 디스플레이7"("Message"=w384) -> ()  [unwired: 9 in, 2 out]
              }
              frame True {
                n169 = Bundle By Name(cluster=w397, "1000원"=TRUE) -> (w395:T2)
                n170 = Unbundle By Name(w392) -> ("재고2"=w394:i32)
                n171 = Unbundle By Name(w400) -> ("잔여금액"=w401:i32)
                n172 = Decrement(x=w394) -> (x-1=w393:i32)
                n173 = Subtract(x=w401, y=1000) -> (x-y=w403:i32)
                n174 = Bundle By Name(cluster=w400, "잔여금액"=w403) -> (w399:cluster{"잔여금액":i32, "카드결제\n금액":i32, "음료가격":i32})
                n175 = Bundle By Name(cluster=w392, "재고2"=w393) -> (w391:T1)
              }
            }
          }
          frame 2 {
            n176 = Unbundle By Name(w407) -> ("잔여금액"=w409:i32)
            n177 = Greater Or Equal?(x=w409, y=1500) -> (x >= y?=w408:bool)
            n178 = case shown="거짓" w408 {
              tunnel: w407 -> [w417 w432]
              tunnel: [T5."대기" T5."음료 주문"] -> w413
              tunnel: w412 -> [w421 w430]
              tunnel: [w421 w428] -> w411
              tunnel: [w417 w427] -> w406
              tunnel: w405 -> [w414 w424]
              tunnel: [w414 w423] -> w404
              frame False {
                n179 = Unbundle By Name(w417) -> ("잔여금액"=w420:i32)
                n180 = Subtract(x=1500, y=w420) -> (x-y=w418:i32)
                n181 = Number To Decimal String(number=w418) -> (decimal integer string=w416:string)  [unwired: 1 in]
                n182 = call "텍스트 만들기5"("Beginning Text"=w416) -> ("Result"=w415:string)  [unwired: 13 in, 1 out]
                n183 = call "사용자에게 메시지 디스플레이9"("Message"=w415) -> ()  [unwired: 9 in, 2 out]
              }
              frame True {
                n184 = Unbundle By Name(w432) -> ("잔여금액"=w433:i32)
                n185 = Unbundle By Name(w424) -> ("재고3"=w426:i32)
                n186 = Bundle By Name(cluster=w430, "1500원"=TRUE) -> (w428:T2)
                n187 = Decrement(x=w426) -> (x-1=w425:i32)
                n188 = Subtract(x=w433, y=1500) -> (x-y=w435:i32)
                n189 = Bundle By Name(cluster=w432, "잔여금액"=w435) -> (w427:cluster{"잔여금액":i32, "카드결제\n금액":i32, "음료가격":i32})
                n190 = Bundle By Name(cluster=w424, "재고3"=w425) -> (w423:T1)
              }
            }
          }
          frame 3 {
            n191 = Unbundle By Name(w439) -> ("잔여금액"=w440:i32)
            n192 = Greater Or Equal?(x=w440, y=2000) -> (x >= y?=w438:bool)
            n193 = case shown="거짓" w438 {
              tunnel: w439 -> [w449 w464]
              tunnel: [w449 w463] -> w445
              tunnel: [T5."대기" T5."음료 주문"] -> w444
              tunnel: w443 -> [w453 w461]
              tunnel: [w453 w459] -> w442
              tunnel: w437 -> [w446 w456]
              tunnel: [w446 w455] -> w436
              frame False {
                n194 = Unbundle By Name(w449) -> ("잔여금액"=w452:i32)
                n195 = Subtract(x=2000, y=w452) -> (x-y=w450:i32)
                n196 = Number To Decimal String(number=w450) -> (decimal integer string=w448:string)  [unwired: 1 in]
                n197 = call "텍스트 만들기6"("Beginning Text"=w448) -> ("Result"=w447:string)  [unwired: 13 in, 1 out]
                n198 = call "사용자에게 메시지 디스플레이6"("Message"=w447) -> ()  [unwired: 9 in, 2 out]
              }
              frame True {
                n199 = Unbundle By Name(w464) -> ("잔여금액"=w465:i32)
                n200 = Unbundle By Name(w456) -> ("재고4"=w458:i32)
                n201 = Bundle By Name(cluster=w461, "2000원"=TRUE) -> (w459:T2)
                n202 = Subtract(x=w465, y=2000) -> (x-y=w467:i32)
                n203 = Decrement(x=w458) -> (x-1=w457:i32)
                n204 = Bundle By Name(cluster=w464, "잔여금액"=w467) -> (w463:cluster{"잔여금액":i32, "카드결제\n금액":i32, "음료가격":i32})
                n205 = Bundle By Name(cluster=w456, "재고4"=w457) -> (w455:T1)
              }
            }
          }
        }
      }
      frame "음료 주문" {
        # "2)"
        # "1)"
        # "주문한 음료가 나오고, 상태 변화 \n1) 음료가 나온 뒤 다음 상태를 결정 하는 케이스들  \n2) 음료의 종류에 따른 선택 후 음료 떨어 지는 동작 시작"
        n206 = Unbundle By Name(w483) -> ("카드"=w477:bool)
        n207 = Unbundle By Name(w480) -> ("잔여금액"=w479:i32)
        n208 = Cluster To Array(cluster=w482) -> (array=w486:bool[])
        n209 = Search 1D Array(1D array=w486, element=TRUE ("원소")) -> (index of element=w484:i32)  [unwired: 1 in]
        n210 = Equal To 0?(x=w479) -> (x = 0?=w471:bool)
        n211 = Select(t=T5."카드", s=w477, f=T5."돈 투입") -> (s? t:f=w473:T5)
        n212 = Select(t=T5."돈 반환", s=w474, f=w473) -> (s? t:f=w470:T5)
        n213 = Select(t=T5."대기", s=w471, f=w470) -> (s? t:f=w468:T5)
        n214 = case shown="1" w484 {
          frame -1, Default {
          }
          frame 0 {
            n215 = while {
              shift-right: [w491] -> _
              shift-left: 0.0 -> [w492]
              stop <- w489 stop-if-true
              n216 = Increment(x=w492) -> (x+1=w491:dbl)
              "콜라뽑음" <- w491
              n217 = Wait Until Next ms Multiple(millisecond multiple=u32 100 ("ms 배수")) -> ()  [unwired: 1 out]
              n218 = Equal?(x=w491, y=10) -> (x = y?=w489:bool)
            }
          }
          frame 1 {
            n219 = while {
              shift-right: [w494] -> _
              shift-left: 0.0 -> [w498]
              stop <- w496 stop-if-true
              n220 = Increment(x=w498) -> (x+1=w494:dbl)
              "사이다 뽑음" <- w494
              n221 = Wait Until Next ms Multiple(millisecond multiple=u32 100 ("ms 배수")) -> ()  [unwired: 1 out]
              n222 = Equal?(x=w494, y=10) -> (x = y?=w496:bool)
            }
          }
          frame 2 {
            n223 = while {
              shift-right: [w500] -> _
              shift-left: 0.0 -> [w504]
              stop <- w502 stop-if-true
              n224 = Increment(x=w504) -> (x+1=w500:dbl)
              "비타민" <- w500
              n225 = Wait Until Next ms Multiple(millisecond multiple=u32 100 ("ms 배수")) -> ()  [unwired: 1 out]
              n226 = Equal?(x=w500, y=10) -> (x = y?=w502:bool)
            }
          }
          frame 3 {
            n227 = while {
              shift-right: [w507] -> _
              shift-left: 0.0 -> [w510]
              stop <- w506 stop-if-true
              n228 = Increment(x=w510) -> (x+1=w507:dbl)
              "파워" <- w507
              n229 = Wait Until Next ms Multiple(millisecond multiple=u32 100 ("ms 배수")) -> ()  [unwired: 1 out]
              n230 = Equal?(x=w507, y=10) -> (x = y?=w506:bool)
            }
          }
        }
      }
      frame "카드" {
        # "3)"
        # "* 카드 사용 법: 카드를 한번 누르게 되면 음료를 선택할 수 있고 음료 선택에 따라 결제 금액이 뜬다. \n카드를 한번 더 누르면 결제 완료가 되고 대기 상태로 돌아 가게 된다.\n1) 카드 한번 더 누른 후 결제 완료 창\n2) 7초간 카드 한번 더 누르지 않을 시, 해당 음료 까지만 계산 완료하고 대기 상태로 바뀜.\n3) 음료에 따라 음료 내려오고, 카드결제 금액 증가"
        n231 = Bundle(cluster=w517, "700원"=w534, "1000원"=w533, "1500원"=w532, "2000원"=w531) -> (w516:T2)
        n232 = Cluster To Array(cluster=w516) -> (array=w530:bool[])
        n233 = Unbundle(w516) -> ("700원"=w515:bool, "1000원"=w514:bool, "1500원"=w513:bool, "2000원"=w512:bool)
        n234 = Search 1D Array(1D array=w530, element=TRUE ("원소")) -> (index of element=w528:i32)  [unwired: 1 in]
        n235 = Compound Arithmetic op=OR ("복합 연산")(w515, w514, w513, w512) -> (w511:bool)
        n236 = case shown="거짓" w519 {
          tunnel: w527 -> [_ w547]
          tunnel: w526 -> [w541 _]
          tunnel: [w536 컨트롤_3."대기"] -> w525
          tunnel: w511 -> [w535 _]
          frame False {
            # "2)"
            n237 = call "경과 시간2"("Time Target (s)"=7.0, "Reset"=w535) -> ("Time has Elapsed"=w540:bool)  [unwired: 10 in, 7 out]
            n238 = Or(x=w540, y=w541) -> (x .or. y?=w539:bool)
            n239 = Select(t=컨트롤_3."대기", s=w539, f=컨트롤_3."카드") -> (s? t:f=w536:T4)
          }
          frame True {
            # "1)"
            n240 = Unbundle By Name(w547) -> ("카드결제\n금액"=w546:i32)
            n241 = Number To Decimal String(number=w546) -> (decimal integer string=w545:string)  [unwired: 1 in]
            n242 = call "텍스트 만들기2"("Beginning Text"=w545) -> ("Result"=w544:string)  [unwired: 13 in, 1 out]
            n243 = call "사용자에게 메시지 디스플레이5"("Message"=w544) -> ()  [unwired: 9 in, 2 out]
          }
        }
        n244 = case shown="0" w528 {
          tunnel: [w549 w555 w570 w585 w600] -> w524
          tunnel: w527 -> [w549 w556 w571 w586 w601]
          tunnel: w521 -> [w548 w551 w566 w581 w596]
          tunnel: [w548 w550 w565 w580 w595] -> w520
          frame -1, Default {
          }
          frame 0 {
            n245 = Unbundle By Name(w551) -> ("재고1"=w553:i32)
            n246 = Unbundle By Name(w556) -> ("카드결제\n금액"=w559:i32)
            n247 = while {
              shift-right: [w560] -> _
              shift-left: 0.0 -> [w564]
              stop <- w562 stop-if-true
              n248 = Increment(x=w564) -> (x+1=w560:dbl)
              n249 = Wait Until Next ms Multiple(millisecond multiple=u32 100 ("ms 배수")) -> ()  [unwired: 1 out]
              n250 = Equal?(x=w560, y=10) -> (x = y?=w562:bool)
              n251 = local write "콜라뽑음"(w560) -> ()
            }
            n252 = Decrement(x=w553) -> (x-1=w552:i32)
            n253 = Bundle By Name(cluster=w551, "재고1"=w552) -> (w550:T1)
            n254 = Add(x=w559, y=700) -> (x+y=w557:i32)
            n255 = Bundle By Name(cluster=w556, "카드결제\n금액"=w557) -> (w555:cluster{"잔여금액":i32, "카드결제\n금액":i32, "음료가격":i32})
          }
          frame 1 {
            n256 = Unbundle By Name(w566) -> ("재고2"=w567:i32)
            n257 = Unbundle By Name(w571) -> ("카드결제\n금액"=w574:i32)
            n258 = while {
              shift-right: [w575] -> _
              shift-left: 0.0 -> [w579]
              stop <- w577 stop-if-true
              n259 = Increment(x=w579) -> (x+1=w575:dbl)
              n260 = Wait Until Next ms Multiple(millisecond multiple=u32 100 ("ms 배수")) -> ()  [unwired: 1 out]
              n261 = local write "사이다 뽑음"(w575) -> ()
              n262 = Equal?(x=w575, y=10) -> (x = y?=w577:bool)
            }
            n263 = Decrement(x=w567) -> (x-1=w568:i32)
            n264 = Bundle By Name(cluster=w566, "재고2"=w568) -> (w565:T1)
            n265 = Add(x=w574, y=1000) -> (x+y=w572:i32)
            n266 = Bundle By Name(cluster=w571, "카드결제\n금액"=w572) -> (w570:cluster{"잔여금액":i32, "카드결제\n금액":i32, "음료가격":i32})
          }
          frame 2 {
            n267 = Unbundle By Name(w581) -> ("재고3"=w583:i32)
            n268 = Unbundle By Name(w586) -> ("카드결제\n금액"=w589:i32)
            n269 = while {
              shift-right: [w590] -> _
              shift-left: 0.0 -> [w594]
              stop <- w592 stop-if-true
              n270 = Increment(x=w594) -> (x+1=w590:dbl)
              n271 = Wait Until Next ms Multiple(millisecond multiple=u32 100 ("ms 배수")) -> ()  [unwired: 1 out]
              n272 = Equal?(x=w590, y=10) -> (x = y?=w592:bool)
              n273 = local write "비타민"(w590) -> ()
            }
            n274 = Decrement(x=w583) -> (x-1=w582:i32)
            n275 = Bundle By Name(cluster=w581, "재고3"=w582) -> (w580:T1)
            n276 = Add(x=w589, y=1500) -> (x+y=w587:i32)
            n277 = Bundle By Name(cluster=w586, "카드결제\n금액"=w587) -> (w585:cluster{"잔여금액":i32, "카드결제\n금액":i32, "음료가격":i32})
          }
          frame 3 {
            n278 = Unbundle By Name(w596) -> ("재고4"=w598:i32)
            n279 = Unbundle By Name(w601) -> ("카드결제\n금액"=w604:i32)
            n280 = while {
              shift-right: [w605] -> _
              shift-left: 0.0 -> [w609]
              stop <- w606 stop-if-true
              n281 = Increment(x=w609) -> (x+1=w605:dbl)
              n282 = Wait Until Next ms Multiple(millisecond multiple=u32 100 ("ms 배수")) -> ()  [unwired: 1 out]
              n283 = Equal?(x=w605, y=10) -> (x = y?=w606:bool)
              n284 = local write "파워"(w605) -> ()
            }
            n285 = Decrement(x=w598) -> (x-1=w597:i32)
            n286 = Bundle By Name(cluster=w596, "재고4"=w597) -> (w595:T1)
            n287 = Add(x=w604, y=2000) -> (x+y=w602:i32)
            n288 = Bundle By Name(cluster=w601, "카드결제\n금액"=w602) -> (w600:cluster{"잔여금액":i32, "카드결제\n금액":i32, "음료가격":i32})
          }
        }
        n289 = Unbundle By Name(w524) -> ("카드결제\n금액"=w523:i32)
        n290 = local write "Display \nMoney"(w523) -> ()
      }
    }
    n291 = Unbundle(w13) -> ("재고1"=w9:i32, "재고2"=w16:i32, "재고3"=w15:i32, "재고4"=w14:i32)
    n292 = Unbundle By Name(w42) -> ("잔여금액"=→"Display \nMoney":i32)
    n293 = Unbundle(w10) -> ("오백원 갯수"=w23:i32, "백원 갯수"=w22:i32)
    n294 = Not Equal To 0?(x=w14) -> (x != 0?=w29:bool)
    n295 = Number To Decimal String(number=w14) -> (decimal integer string=w28:string)  [unwired: 1 in]
    n296 = Number To Decimal String(number=w16) -> (decimal integer string=w34:string)  [unwired: 1 in]
    n297 = Number To Decimal String(number=w15) -> (decimal integer string=w31:string)  [unwired: 1 in]
    n298 = Not Equal To 0?(x=w16) -> (x != 0?=w35:bool)
    n299 = Number To Decimal String(number=w9) -> (decimal integer string=w18:string)  [unwired: 1 in]
    n300 = Number To Decimal String(number=w23) -> (decimal integer string=→"오백원 갯수":string)  [unwired: 1 in]
    n301 = Not Equal To 0?(x=w9) -> (x != 0?=w36:bool)
    n302 = Not Equal To 0?(x=w15) -> (x != 0?=w32:bool)
    n303 = Select(t=w28, s=w29, f="매진") -> (s? t:f=→"파워에이드 재고":string)
    n304 = Number To Decimal String(number=w22) -> (decimal integer string=→"백원 갯수":string)  [unwired: 1 in]
    n305 = Select(t=w34, s=w35, f="매진" ("t")) -> (s? t:f=→"사이다 재고":string)
    n306 = Select(t=w31, s=w32, f="매진") -> (s? t:f=→"비타민 워터 재고":string)
    n307 = Select(t=w18, s=w36, f="매진" ("t")) -> (s? t:f=→"콜라 재고":string)
  }
